vi "Test Assign Value.vi"() -> ()   [LabVIEW 2021]
uses:
  Source/Variables/Support/Bool/Support/Init_Simple_Var.vi
  Source/Abs_Types/Boolean/Static Read.vi
  Source/Variables/Support/Bool/Var_Bool.lvclass
  C:/TSA/LV_Abstract/Source/Abs_Types/Boolean/Abs_Boolean.lvclass
  Source/Abs_Types/Boolean/Abs_Boolean.lvclass
  C:/Program Files (x86)/National Instruments/LabVIEW 2021/vi.lib/TSA/Abstract Data Classes/Abs_Types/Value/Abs_Value.lvclass
  Source/Constants/Support/Bool/Bool.vi
  Source/Constants/Support/Bool/Const_Bool.lvclass
  C:/Program Files (x86)/National Instruments/LabVIEW 2021/vi.lib/TSA/Abstract Data Classes/Abs_Types/Type/Abs_Type.lvclass
  C:/TSA/LV_Abstract/Source/Variables/Support/Bool/Var_Bool.lvclass
panel:
  out "Boolean 2":bool
  out "Boolean":bool
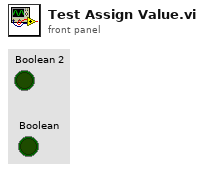
[diagram p1: front panel]
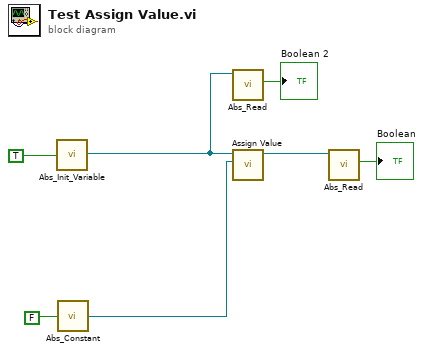
[diagram p0: block diagram]
diagram:
  n1 = call-poly "Abs_Init_Variable.vi"("Value"=TRUE) -> ("Var"=w1:refnum<class "Var_Bool.lvclass">)  [unwired: 4 in]
  n2 = call-poly "Abs_Constant.vi"("Boolean"=FALSE) -> ("Abs_Boolean.lvclass"=w7:refnum<class "Abs_Boolean.lvclass">)  [unwired: 4 in]
  n3 = call-poly "Abs_Read.vi"("Abs_Boolean in"=w1) -> ("Boolean"=→"Boolean 2":bool)  [unwired: 8 in, 2 out]
  n4 = call-dynamic "Assign Value.vi"("Assigned Value"=w7, "Abs_Boolean in"=w1) -> ("Abs_Boolean out"=w6:refnum<class "Var_Bool.lvclass">)  [unwired: 8 in, 1 out]
  n5 = call-poly "Abs_Read.vi"("Abs_Boolean in"=w6) -> ("Boolean"=→"Boolean":bool)  [unwired: 8 in, 2 out]
